vi "XL320_Capture Motor Positions.vi"(1 "Motor List (Numeric)":u8[](array[numeric]), 2 "Com Port":refnum<visa-resource-name>) -> (0 "Positions (deg)":dbl[](array[numeric]))   [LabVIEW 2015]
doc: "Queries all of the motors in <B>Motor List</B> and returns their respective <B>Positions</B>."
uses:
  <instrlib>/Dynamixel XL320/Dynamixel XL320.lvlib
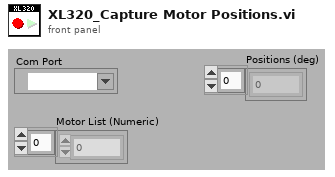
[diagram p1: front panel]
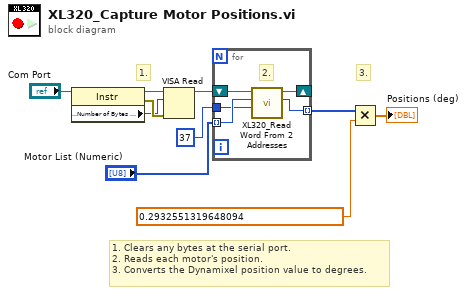
[diagram p0: block diagram]
diagram:
  # "3."
  # "1."
  # "1. Clears any bytes at the serial port.\n2. Reads each motor's position.\n3. Converts the Dynamixel position value to degrees."
  n1 = property class="Instr"(reference="Com Port") -> (reference out=w4:refnum<visa-resource-name>, error out=w6:errorcluster, "Serial Settings:Number of Bytes at Serial Port"=w5:u32)  [unwired: 1 in]
  n2 = VISA Read(VISA resource name=w4, byte count=w5, error in (no error)=w6) -> (VISA resource name out=w3:refnum<visa-resource-name>)  [unwired: 3 out]
  n3 = for {
    tunnel: [w11] -> w1 mode=indexing
    shift-right: [w12] -> _
    shift-left: w3 -> [w15]
    tunnel: "Motor List (Numeric)" -> [w14] mode=indexing
    tunnel: u16 37 -> [w13]
    # "2."
    n4 = call <instrlib>:"XL320_Read Word From 2 Addresses.vi"("Address number (0)"=w13, "Motor ID (0)"=w14, "VISA resource name"=w15) -> ("Data"=w11:u16, "VISA resource name out"=w12:refnum<visa-resource-name>)  [unwired: 6 in, 1 out]
  }
  n5 = Multiply(x=w1, y=0.2932551319648094) -> (x*y=→"Positions (deg)":dbl[])
